vi "TWM Client Cmd Identify.vi"(5 "timeout [ms]":i32=5000, 7 "end of packet key":string="TWM:command:EndOfPacket", 8 "error in":errorcluster, 11 "handle":i32) -> (0 "error out":errorcluster, 1 "aux idns":string[](array[string]), 2 "channel idns":string[](array[string]), 3 "handle out":i32)   [LabVIEW 2020, in "TWM Client.lvlib"]
doc: "Write Identify command packet to TWM server. Wait for answer. Parse and return data."
uses:
  TWM Client.lvlib
  Get 1D String.vi
  <vilib>/Utility/error.llb/Error Cluster From Error Code.vi
  <vilib>/ErrorRing/Error Ring.xnode
  infolib.lvlib
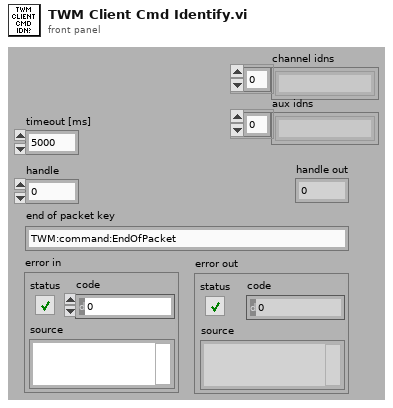
[diagram p1: front panel]
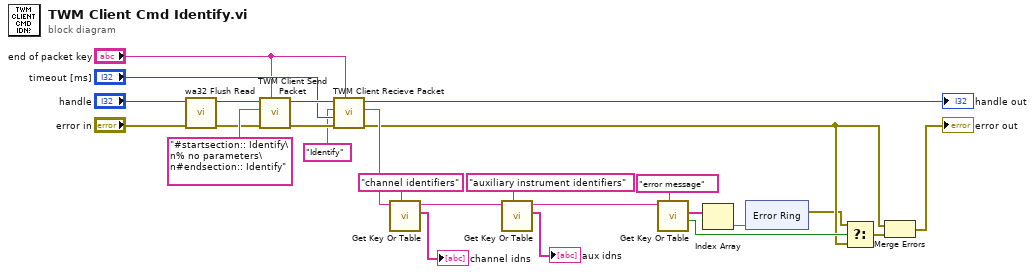
[diagram p0: block diagram]
diagram:
  n1 = call "wa32 Flush Read.vi"("error in"="error in", "handle"="handle") -> ("error out"=w3:errorcluster, "handle out"=w2:i32)  [unwired: 7 in, 1 out]
  n2 = call "TWM Client Send Packet.vi"("end of packet key"="end of packet key", "error in"=w3, "command string"="#startsection:: Identify\n% no parameters\n#endsection:: Identify", "handle"=w2) -> ("error out"=w25:errorcluster, "handle out"=w24:i32)  [unwired: 6 in]
  n3 = call "TWM Client Recieve Packet.vi"("end of packet key"="end of packet key", "error in"=w25, "timeout [ms] (5000 ms)"="timeout [ms]", "message header (empty)"="Identify", "handle in"=w24) -> ("error out"=w6:errorcluster, "message data"=w19:string, "handle out"=→"handle out":i32)  [unwired: 4 in]
  n4 = call-poly "Get Key Or Table.vi"("key description"="channel identifiers", "info data"=w19) -> ("value"=→"channel idns":string[], "info data out"=w16:string)  [unwired: 6 in, 2 out]
  n5 = call-poly "Get Key Or Table.vi"("key description"="auxiliary instrument identifiers", "info data"=w16) -> ("value"=→"aux idns":string[], "info data out"=w12:string)  [unwired: 6 in, 2 out]
  n6 = call-poly "Get Key Or Table.vi"("key description"="error message", "info data"=w12) -> ("key found?"=w9:bool, "value"=w8:string[])  [unwired: 6 in, 2 out]
  n7 = Index Array(array=w8) -> (element=w7:string)  [unwired: 1 in]
  n8 = xnode "Error Ring"("parameter 0"=w7) -> ("error out"=w5:errorcluster)
  n9 = Select(t=w5, s=w9, f=w6) -> (s? t:f=w11:errorcluster)
  n10 = Merge Errors(w6, w11) -> (→"error out":errorcluster)
